vi "Configure Level.vi"(0 "VISA resource name":refnum<visa-resource-name>, 5 "Channel (0: Channel 1)":u16(ring) items=["Channel 1", "Channel 2"], 7 "Level (0:high)":u16(ring) items=["High", "Low"], 9 "Level (V)":dbl=1.0, 11 "error in (no error)":errorcluster) -> (4 "VISA resource name out":refnum<visa-resource-name>, 15 "error out":errorcluster)   [LabVIEW 2019]
doc: "Selects the waveform shape, frequency, amplitude, offset, and phase \nfor a standard waveform."
uses:
  <userlib>/Tektronix AFG 3000 Series/Tektronix AFG 3000 Series.lvlib
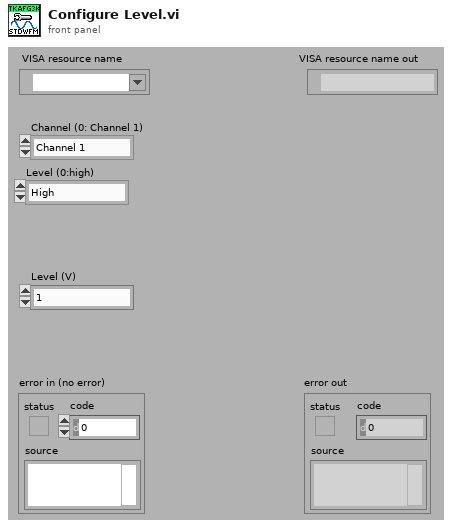
[diagram p1: front panel]
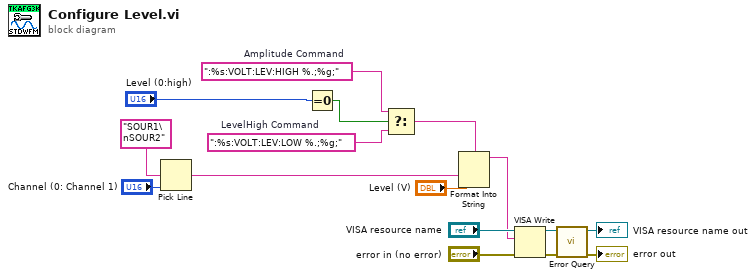
[diagram p0: block diagram]
diagram:
  w5 = ":%s:VOLT:LEV:LOW %.;%g;"  # LevelHigh Command
  w6 = ":%s:VOLT:LEV:HIGH %.;%g;"  # Amplitude Command
  n1 = Pick Line(multi-line string="SOUR1\nSOUR2" ("string (\"\")"), line index="Channel (0: Channel 1)") -> (output string=w7:string)  [unwired: 1 in]
  n2 = Equal To 0?(x="Level (0:high)") -> (x = 0?=w2:bool)
  n3 = Select(t=w6, s=w2, f=w5) -> (s? t:f=w4:string)
  n4 = Format Into String(format string=w4, w7, "Level (V)") -> (resulting string=w3:string)  [unwired: 2 in, 1 out]
  n5 = VISA Write(VISA resource name="VISA resource name", write buffer=w3, error in (no error)="error in (no error)") -> (VISA resource name out=w12:refnum<visa-resource-name>, error out=w11:errorcluster)  [unwired: 1 out]
  n6 = call <userlib>:"Error Query.vi"("error in (no error)"=w11, "VISA resource name"=w12) -> ("error out"=→"error out":errorcluster, "VISA resource name out"=→"VISA resource name out":refnum<visa-resource-name>)  [unwired: 6 in, 2 out]
